vi "RawOdometryAccumalator.vi"(0 "Position":dbl, 1 "Initial Offset":cluster{"X":dbl, "Y":dbl}, 2 "Heading":dbl) -> (5 "X":dbl, 6 "Y":dbl)   [LabVIEW 2018]
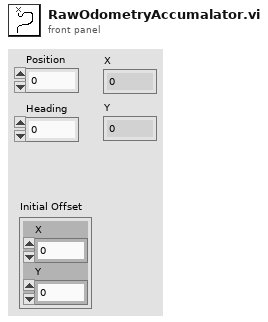
[diagram p1: front panel]
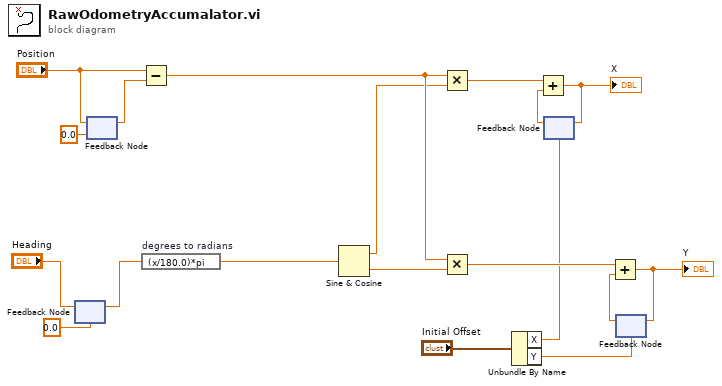
[diagram p0: block diagram]
diagram:
  n1 = feedback #1(0.0 ("Heading")) -> (w1:dbl)
  n2 = feedback-in #1("Heading") -> ()
  n3 = feedback-in #2("Position") -> ()
  n4 = feedback #2(0.0 ("Position")) -> (w17:dbl)
  n5 = Subtract(x="Position", y=w17) -> (x-y=w15:dbl)
  n6 = expression code="(x/180.0)*pi" "degrees to radians"(w1) -> (w8:dbl)
  n7 = Sine & Cosine(0:w8) -> (1:w6:dbl, 2:w7:dbl)
  n8 = Multiply(x=w15, y=w6) -> (x*y=w14:dbl)
  n9 = Multiply(x=w15, y=w7) -> (x*y=w13:dbl)
  n10 = Unbundle By Name("Initial Offset") -> ("X"=w4:dbl, "Y"=w3:dbl)
  n11 = feedback #3(w4) -> (w12:dbl)
  n12 = Add(x=w14, y=w12) -> (x+y=w9:dbl)
  "X" <- w9
  n13 = feedback-in #3(w9) -> ()
  n14 = feedback #4(w3) -> (w11:dbl)
  n15 = Add(x=w13, y=w11) -> (x+y=w10:dbl)
  "Y" <- w10
  n16 = feedback-in #4(w10) -> ()
